vi "Write Array of VacuumLine Objs.vi"(10 "Array of VacuumLine Objs":refnum<class "VacuumLine.lvclass">[](array[class]), 11 "VacuumLines in":refnum<class "VacuumLines.lvclass">) -> (3 "VacuumLines out":refnum<class "VacuumLines.lvclass">)   [LabVIEW 2016, in "Hardware.lvlib" / "VacuumLine.lvlib" / "VacuumLines.lvclass"]
uses:
  <userlib>/Common Components/Hardware/Abstract System/VacuumLine/VacuumLines/VacuumLines.lvclass
  <userlib>/Common Components/Hardware/Abstract System/VacuumLine/VacuumLine/VacuumLine.lvclass
  <userlib>/Common Components/Hardware/Abstract System/VacuumLine/VacuumLines/VacuumLines.lvclass/VacuumLines.ctl
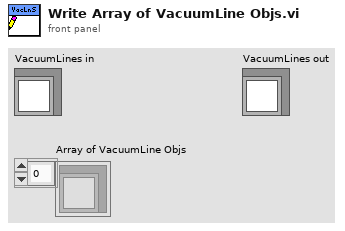
[diagram p1: front panel]
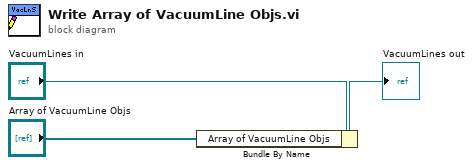
[diagram p0: block diagram]
diagram:
  n1 = Bundle By Name(cluster="VacuumLines in", "Array of VacuumLine Objs"="Array of VacuumLine Objs") -> (→"VacuumLines out":refnum<class "VacuumLines.lvclass">)
